vi "HandleStop.vi"(8 "error in (no error)":errorcluster, 11 "Acquisition in":refnum<class "Acquisition.lvclass">) -> (0 "error out":errorcluster, 2 "stop?":bool, 3 "Acquisition out":refnum<class "Acquisition.lvclass">)   [LabVIEW 2018, in "Acquisition.lvclass"]
uses:
  Acquisition.lvclass
  C:/Users/devstaff/sparc4/s4gui/Versao ZeroMQ REQ-REP/SPARC4_GUI -v1.0.0/Server/Server.lvclass
  Server/Server.lvclass/Server.ctl
  Acquisition.lvclass/Acquisition.ctl
  Channel/Channel.lvclass
  Interface/Interface.lvclass
  Server/Server.lvclass
  StateMachine/State Machine.lvclass
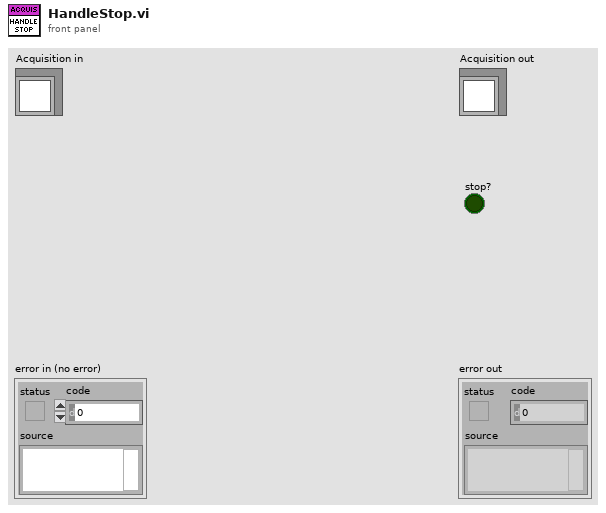
[diagram p1: front panel]
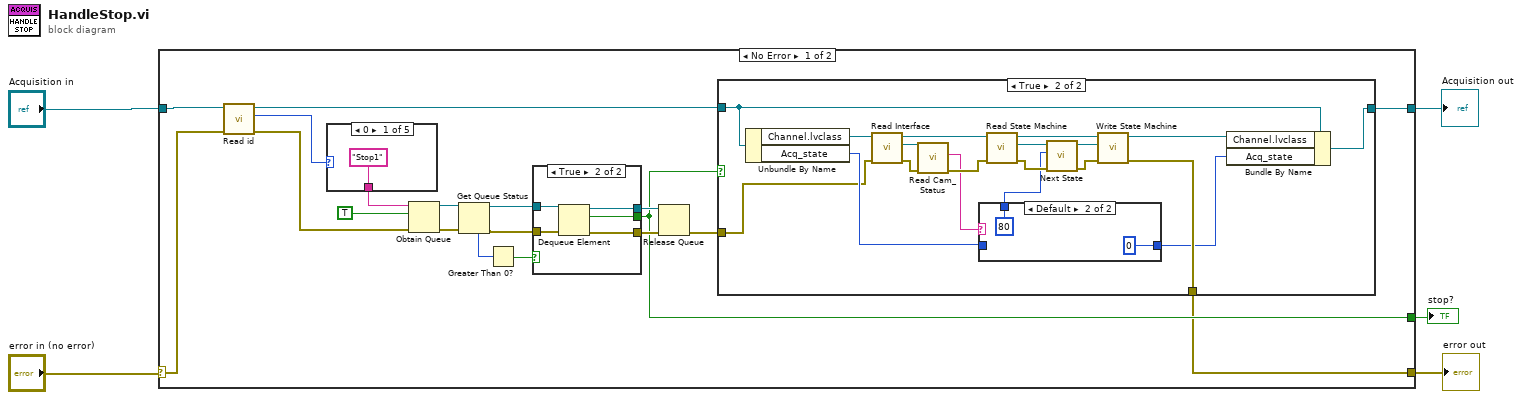
[diagram p0: block diagram]
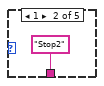
[diagram p2: hidden frame]
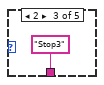
[diagram p3: hidden frame]
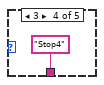
[diagram p4: hidden frame]
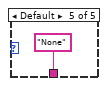
[diagram p5: hidden frame]
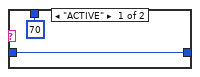
[diagram p7: hidden frame]
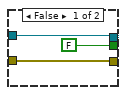
[diagram p8: hidden frame]
diagram:
  n1 = case shown="No Error" "error in (no error)" {
    selector: "error in (no error)" -> [w7 w64]
    tunnel: [w8 w64] -> w3
    tunnel: [w24 w63] -> w2
    tunnel: "Acquisition in" -> [w23 w63]
    tunnel: [w11 _] -> w1
    frame No Error {
      n2 = call "Read id.vi"("error in (no error)"=w7, "Server in"=w23) -> ("error out"=w6:errorcluster, "id"=w10:u32, "Server out"=w22:refnum<class "Acquisition.lvclass">)  [unwired: 7 in]
      n3 = case shown="0" w10 {
        tunnel: ["Stop1" ("name (unnamed)") "Stop2" ("name (unnamed)") "Stop3" ("name (unnamed)") "Stop4" ("name (unnamed)") "None" ("name (unnamed)")] -> w21
        frame 0 {
        }
        frame 1 {
        }
        frame 2 {
        }
        frame 3 {
        }
        frame Default {
        }
      }
      n4 = Obtain Queue(name (unnamed)=w21, element data type=TRUE, error in (no error)=w6) -> (queue out=w18:refnum<queue>, error out=w19:errorcluster)  [unwired: 2 in, 1 out]
      n5 = Get Queue Status(queue=w18, error in (no error)=w19) -> (queue out=w15:refnum<queue>, error out=w14:errorcluster, # elements in queue=w17:i32)  [unwired: 1 in, 5 out]
      n6 = Greater Than 0?(x=w17) -> (x > 0?=w16:bool)
      n7 = case shown="True" w16 {
        tunnel: w15 -> [w56 w61]
        tunnel: w14 -> [w55 w62]
        tunnel: [FALSE w60] -> w11
        tunnel: [w56 w59] -> w13
        tunnel: [w55 w58] -> w12
        frame False {
        }
        frame True {
          n8 = Dequeue Element(queue=w61, error in (no error)=w62) -> (queue out=w59:refnum<queue>, element=w60:bool, error out=w58:errorcluster)  [unwired: 1 in, 1 out]
        }
      }
      n9 = Release Queue(queue=w13, error in (no error)=w12) -> (error out=w9:errorcluster)  [unwired: 1 in, 2 out]
      n10 = case shown="True" w11 {
        tunnel: [w31 w50] -> w24
        tunnel: w22 -> [w31 w49]
        tunnel: w9 -> [w30 w37]
        tunnel: [w30 w42] -> w8
        frame False {
        }
        frame True {
          n11 = Unbundle By Name(w49) -> ("Channel.lvclass"=w36:refnum<class "Channel.lvclass">, "Acq_state"=w38:u32)
          n12 = call-dynamic "Read Interface.vi"("error in (no error)"=w37, "Channel in"=w36) -> ("error out"=w40:errorcluster, "Interface.lvclass"=w41:refnum<class "Interface.lvclass">, "Channel out"=w35:refnum<class "Channel.lvclass">)  [unwired: 7 in]
          n13 = call-dynamic "Read Cam_Status.vi"("error in (no error)"=w40, "Interface in"=w41) -> ("error out"=w34:errorcluster, "Cam_Status"=w32:string)  [unwired: 7 in, 1 out]
          n14 = case shown="Default" w32 {
            tunnel: [70 80] -> w33
            tunnel: [w51 u32 0] -> w39
            tunnel: w38 -> [w51 _]
            frame "ACTIVE" {
            }
            frame Default {
            }
          }
          n15 = call-dynamic "Read State Machine.vi"("error in (no error)"=w34, "Device in"=w35) -> ("error out"=w47:errorcluster, "State Machine.lvclass"=w48:refnum<class "State Machine.lvclass">, "Device out"=w45:refnum<class "Channel.lvclass">)  [unwired: 7 in]
          n16 = call "Next State.vi"("error in (no error)"=w47, "New_State"=w33, "State Machine in"=w48) -> ("error out"=w44:errorcluster, "State Machine out"=w46:refnum<class "State Machine.lvclass">)  [unwired: 7 in]
          n17 = call-dynamic "Write State Machine.vi"("error in (no error)"=w44, "State Machine.lvclass"=w46, "Device in"=w45) -> ("error out"=w42:errorcluster, "Device out"=w43:refnum<class "Channel.lvclass">)  [unwired: 7 in]
          n18 = Bundle By Name(cluster=w49, "Channel.lvclass"=w43, "Acq_state"=w39) -> (w50:refnum<class "Acquisition.lvclass">)
        }
      }
    }
    frame Error {
    }
  }
  "error out" <- w3
  "Acquisition out" <- w2
  "stop?" <- w1
